vi "GT_Stop.vi"(6 "Stop Style":u16(ring) items=["Smooth Stop", "Abrupt Stop"], 8 "Axis Map":T2, 9 "Axis Config":cluster{"Axis x":T1, "Axis y":T1, "Axis z":T1}={"Axis x"=1, "Axis y"=2, "Axis z"=3} {"Axis z" items=["Axis Control"=0, "Axis 1"=1, "Axis 2"=2, "Axis 3"=3, "Axis 4"=4, "Axis 5"=5, "Axis 6"=6, "Axis 7"=7, "Axis 8"=8, "Vector Space Control"=16, "Vector Space 1"=17, "Vector Space 2"=18, "Vector Space 3"=19, "Vector Space 4"=20]; "Axis y" items=["Axis Control"=0, "Axis 1"=1, "Axis 2"=2, "Axis 3"=3, "Axis 4"=4, "Axis 5"=5, "Axis 6"=6, "Axis 7"=7, "Axis 8"=8, "Vector Space Control"=16, "Vector Space 1"=17, "Vector Space 2"=18, "Vector Space 3"=19, "Vector Space 4"=20]; "Axis x" items=["Axis Control"=0, "Axis 1"=1, "Axis 2"=2, "Axis 3"=3, "Axis 4"=4, "Axis 5"=5, "Axis 6"=6, "Axis 7"=7, "Axis 8"=8, "Vector Space Control"=16, "Vector Space 1"=17, "Vector Space 2"=18, "Vector Space 3"=19, "Vector Space 4"=20]}, 10 "Axis in":T1=1 items=["Axis Control"=0, "Axis 1"=1, "Axis 2"=2, "Axis 3"=3, "Axis 4"=4, "Axis 5"=5, "Axis 6"=6, "Axis 7"=7, "Axis 8"=8, "Vector Space Control"=16, "Vector Space 1"=17, "Vector Space 2"=18, "Vector Space 3"=19, "Vector Space 4"=20], 11 "rtn_In":cluster{"rtn":i16, "Func":string}) -> (2 "Axis out":T1=1 items=["Axis Control"=0, "Axis 1"=1, "Axis 2"=2, "Axis 3"=3, "Axis 4"=4, "Axis 5"=5, "Axis 6"=6, "Axis 7"=7, "Axis 8"=8, "Vector Space Control"=16, "Vector Space 1"=17, "Vector Space 2"=18, "Vector Space 3"=19, "Vector Space 4"=20], 3 "rtn_Out":cluster{"rtn":i16, "Func":string})   [LabVIEW 2014]
uses:
  <vilib>/Motion/FlexMotion/CustomControls/CustomControls.llb/AxisOrVectorSpaceControl To Control.flx
  VC6/gts.dll
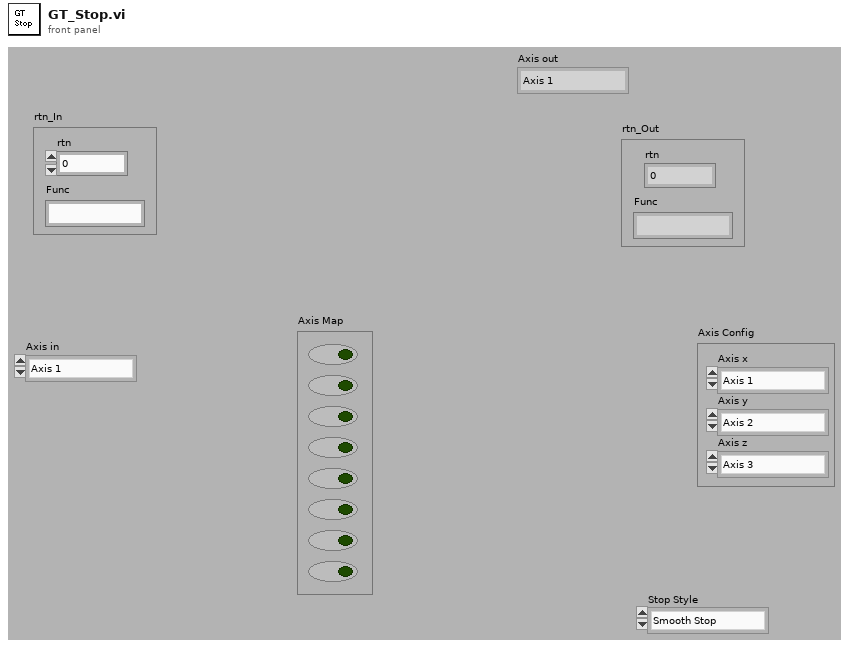
[diagram p1: front panel]
types:
  T1 = typedef "AxisOrVectorSpaceControl To Control.flx" = u16
  T2 = cluster{"Axis1":bool, "Axis2":bool, "Axis3":bool, "Axis4":bool, "Axis5":bool, "Axis6":bool, "Axis7":bool, "Axis8":bool}
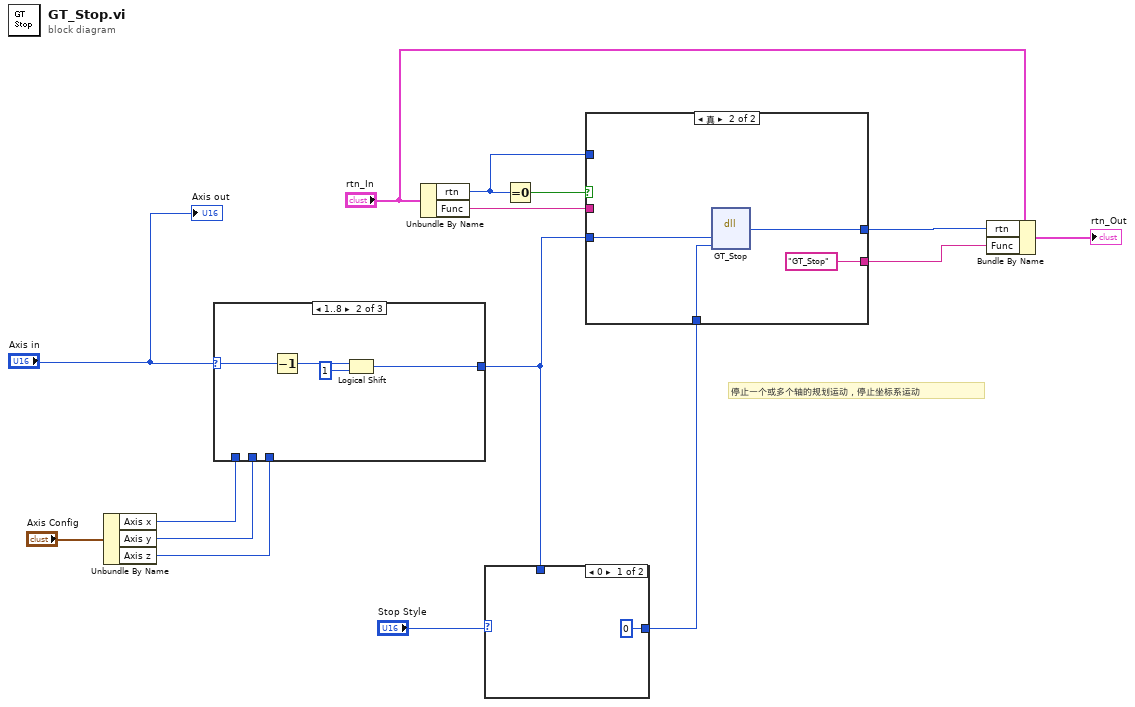
[diagram p0: block diagram]
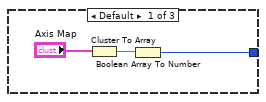
[diagram p3: hidden frame]
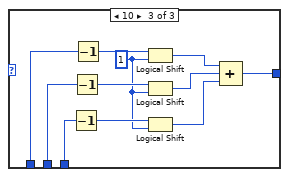
[diagram p4: hidden frame]
diagram:
  # "停止一个或多个轴的规划运动，停止坐标系运动"
  n1 = Unbundle By Name("Axis Config") -> ("Axis x"=w10:T1, "Axis y"=w9:T1, "Axis z"=w8:T1)
  n2 = case shown="1..8" "Axis in" {
    selector: "Axis in" -> [_ w22 _]
    tunnel: [w16 w19 w23] -> w1
    tunnel: w10 -> [_ _ w32]
    tunnel: w9 -> [_ _ w30]
    tunnel: w8 -> [_ _ w28]
    frame Default {
      n3 = Cluster To Array(cluster="Axis Map") -> (array=w17:bool[])
      n4 = Boolean Array To Number(Boolean array=w17) -> (number=w16:u32)
    }
    frame 1..8 {
      n5 = Decrement(x=w22) -> (x-1=w21:T1)
      n6 = Logical Shift(y=w21, x=1) -> (x << y=w19:i32)
    }
    frame 10 {
      w27 = 1
      n7 = Decrement(x=w28) -> (x-1=w29:T1)
      n8 = Decrement(x=w30) -> (x-1=w31:T1)
      n9 = Decrement(x=w32) -> (x-1=w33:T1)
      n10 = Logical Shift(y=w33, x=w27) -> (x << y=w26:i32)
      n11 = Logical Shift(y=w31, x=w27) -> (x << y=w25:i32)
      n12 = Logical Shift(y=w29, x=w27) -> (x << y=w24:i32)
      n13 = Compound Arithmetic op=ADD(w26, w25, w24) -> (w23:i32)
    }
  }
  n14 = Unbundle By Name("rtn_In") -> ("rtn"=w6:i16, "Func"=w5:string)
  n15 = case shown="0" "Stop Style" {
    tunnel: [u32 0 w35] -> w2
    tunnel: w1 -> [_ w35]
    frame 0 {
    }
    frame 1, Default {
    }
  }
  n16 = Equal To 0?(x=w6) -> (x = 0?=w15:bool)
  n17 = case shown="真" w15 {
    tunnel: [w37 w41] -> w12
    tunnel: w1 -> [_ w40]
    tunnel: [w36 "GT_Stop" ("Func")] -> w7
    tunnel: w6 -> [w37 _]
    tunnel: w5 -> [w36 _]
    tunnel: w2 -> [_ w38]
    frame False {
    }
    frame True {
      n18 = dll-call lib="PTH2Fabs DNewGTS AC-800LWin7版源程序-20170926gts85VC6gts.dll" fn="GT_Stop"("Mask"=w40, "option"=w38) -> ("rtn"=w41:i16)  [unwired: 5 in, 2 out]
    }
  }
  n19 = Bundle By Name(cluster="rtn_In", "rtn"=w12, "Func"=w7) -> (→"rtn_Out":cluster{"rtn":i16, "Func":string})
  "Axis out" <- "Axis in"
